vi "Auto Power Spectrum.vi"(2 "dt":dbl=1.0 format="%0.2f", 3 "Signal (V)":dbl[](array[numeric])) -> (0 "df":dbl format="%0.2f", 1 "Power Spectrum (V^2 rms)":dbl[](array[numeric]))   [LabVIEW 2017, in "NI_AALPro.lvlib"]
doc: "Computes the single-sided, scaled, auto power spectrum of a time-domain signal."
uses:
  <vilib>/Analysis/NI_AALPro.lvlib
  <vilib>/Analysis/2dsp.llb/Power Spectrum (DBL).vi
panel:
  # "Auto Power Spectrum"
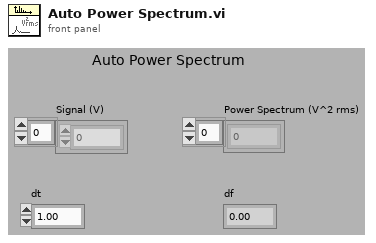
[diagram p1: front panel]
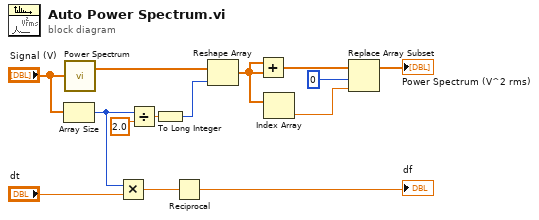
[diagram p0: block diagram]
diagram:
  n1 = Array Size(array="Signal (V)") -> (size(s)=w11:i32)
  n2 = call-poly <vilib>:"Power Spectrum.vi"("X"="Signal (V)") -> ("Power Spectrum"=w7:dbl[])  [unwired: 1 out]
  n3 = Multiply(x=w11, y="dt") -> (x*y=w12:dbl)
  n4 = Divide(x=w11, y=2.0) -> (x/y=w8:dbl)
  n5 = To Long Integer(number=w8) -> (32bit integer=w6:i32)
  n6 = Reciprocal(x=w12) -> (1/x=→"df":dbl)
  n7 = Reshape Array(w7, w6) -> (w5:dbl[])
  n8 = Add(x=w5, y=w5) -> (x+y=w4:dbl[])
  n9 = Index Array(array=w5) -> (element=w3:dbl)  [unwired: 1 in]
  n10 = Replace Array Subset(array=w4, new element=w3, index=0) -> (→"Power Spectrum (V^2 rms)":dbl[])
